vi "clearpath_set_differential_controls.vi"(0 "ClearpathComm":T1, 1 "Controls Cluster":T2) -> ()   [LabVIEW 2012, in "clearpath_interface.lvlib"]
doc: "Formats a Set Differential Control Constants command (0x201) to override the built-in control constants, given speeds in m/s and accelerations in m/s^2. Use with caution, and retrieve the current constants for reference before overriding. A \"D\" value of 0 is recommended. Resetting the processor or power cycling the platform will reset the constants to default. Uses the onboard Clearpath library to perform the actual message formatting."
uses:
  clearpath_interface.lvlib
  cwrap_crio.dll
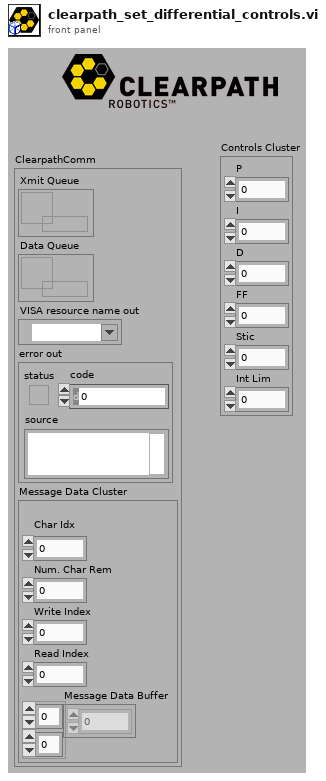
[diagram p1: front panel]
types:
  T1 = cluster{"Xmit Queue":refnum<queue>, "Data Queue":refnum<queue>, "VISA resource name out":refnum<visa-resource-name>, "error out":errorcluster, "Message Data Cluster":cluster{"\nChar Idx":u8, "Num. Char Rem":u8, "Write Index":u8, "Read Index":u8, "Message Data Buffer":u8[][]}}
  T2 = cluster{"P":dbl, "I":dbl, "D":dbl, "FF":dbl, "Stic":dbl, "Int Lim":dbl}
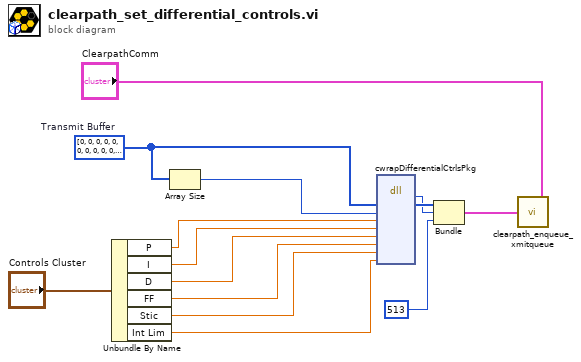
[diagram p0: block diagram]
diagram:
  w13 = u8[] [0, 0, 0, 0, 0, 0, 0, 0, 0, 0, 0, 0, 0, 0, 0, 0, 0, 0, 0, 0, 0, 0, 0, 0, 0, 0, 0, 0, 0, 0, 1, 0, 0, 0, 5, 0, 0, 0, 0, 0, 0]  # Transmit Buffer
  n1 = Unbundle By Name("Controls Cluster") -> ("P"=w11:dbl, "I"=w8:dbl, "D"=w7:dbl, "FF"=w9:dbl, "Stic"=w6:dbl, "Int Lim"=w10:dbl)
  n2 = Array Size(array=w13) -> (size(s)=w14:i32)
  n3 = dll-call lib="C:/Users/cartersm/Documents/GitHub/IGVC-2013/Code/Project 1.0/Motors/Husky/cwrap_cRIO.*" fn="cwrapDifferentialCtrlsPkg"("buf"=w13, "buf_size"=w14, "p"=w11, "i"=w8, "d"=w7, "ffwd"=w9, "stic"=w6, "i_lim"=w10) -> ("return type"=w4:i32, "buf"=w5:u8[])  [unwired: 10 in, 2 out]
  n4 = Bundle("buf"=w5, "return type"=w4, 513) -> (w1:cluster{"buf":u8[], "return type":i32, i32})  [unwired: 1 in]
  n5 = call "clearpath_enqueue_xmitqueue.vi"("ClearpathComm"="ClearpathComm", "Cluster"=w1) -> ()
